vi "Configure DAC Range.vi"(4 "DAC Channel":u32, 5 "start label":string, 6 "Full scale range":u32=10, 7 "waveform name":string, 8 "error in":errorcluster, 11 "Digital session":refnum<k15>) -> (0 "error out":errorcluster, 3 "Digital session out":refnum<k15>)   [LabVIEW 2021]
uses:
  <instrlib>/niDigital/niDigital.llb/niDigital Write Source Waveform (Broadcast U32).vi
  <instrlib>/niDigital/niDigital.llb/niDigital Burst Pattern (Pass Fail).vi
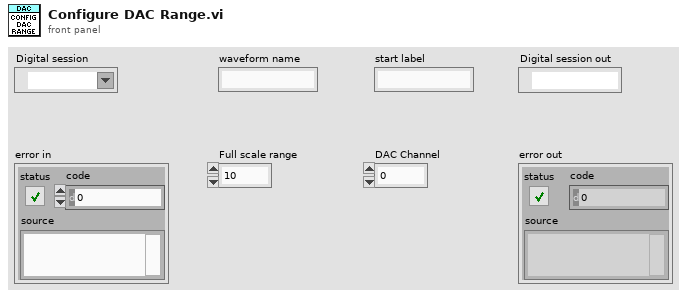
[diagram p1: front panel]
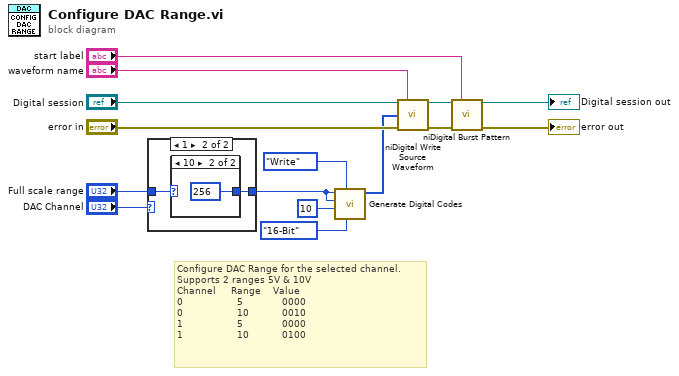
[diagram p0: block diagram]
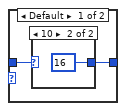
[diagram p2: hidden frame]
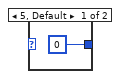
[diagram p3: hidden frame]
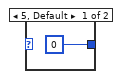
[diagram p4: hidden frame]
diagram:
  # "Configure DAC Range for the selected channel.\nSupports 2 ranges 5V & 10V\nChannel     Range    Value\n0                  5             0000\n0                  10           0010\n1                  5             0000\n1                  10           0100"
  n1 = case shown="1" "DAC Channel" {
    tunnel: [w16 w20] -> w1
    tunnel: "Full scale range" -> [w17 w21]
    frame Default {
      n2 = case shown="10" w17 {
        tunnel: [u16 0 u16 16] -> w16
        frame 5, Default {
        }
        frame 10 {
        }
      }
    }
    frame 1 {
      n3 = case shown="10" w21 {
        tunnel: [u16 0 u16 256] -> w20
        frame 5, Default {
        }
        frame 10 {
        }
      }
    }
  }
  n4 = call "Generate Digital Codes.vi"("Input Code Bit"=enum16{"16-Bit", "12-Bit"}."16-Bit", "Command"=enum16{"Read", "Write"}."Write", "Address"=u8 10, "End code"=w1, "Start code"=w1) -> ("Digital commands"=w3:i16[])  [unwired: 4 in, 2 out]
  n5 = call-poly <instrlib>:"niDigital Write Source Waveform.vi"("instrument handle"="Digital session", "waveform name"="waveform name", "waveform data"=w3, "error in"="error in") -> ("instrument handle out"=w5:refnum<k15>, "error out"=w4:errorcluster)  [unwired: 10 in]
  n6 = call-poly <instrlib>:"niDigital Burst Pattern.vi"("instrument handle"=w5, "start label"="start label", "error in"=w4) -> ("instrument handle out"=→"Digital session out":refnum<k15>, "error out"=→"error out":errorcluster)  [unwired: 10 in, 1 out]
